vi "Write mode ref.vi"(8 "error in (no error)":errorcluster caption="에러 입력(에러 없음)", 10 "mode ref":refnum<vi>, 11 "Haptic IC 입력":refnum<class "Haptic IC.lvclass">) -> (0 "error out":errorcluster caption="에러 출력", 3 "Haptic IC 출력":refnum<class "Haptic IC.lvclass">)   [LabVIEW 2020, in "Haptic IC.lvclass"]
uses:
  Haptic IC.lvclass
  Haptic IC.lvclass/Haptic IC.ctl
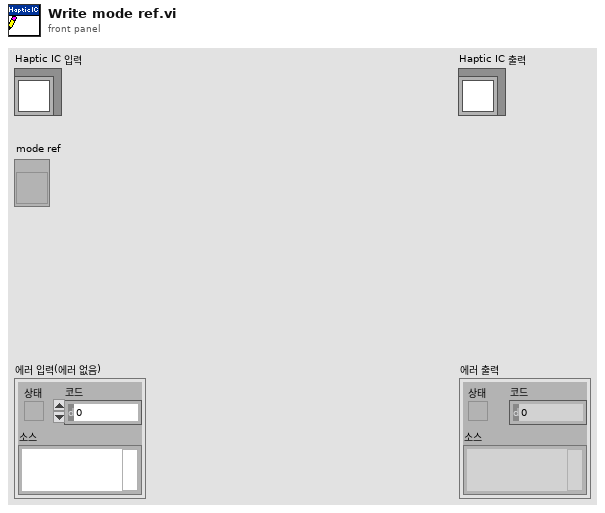
[diagram p1: front panel]
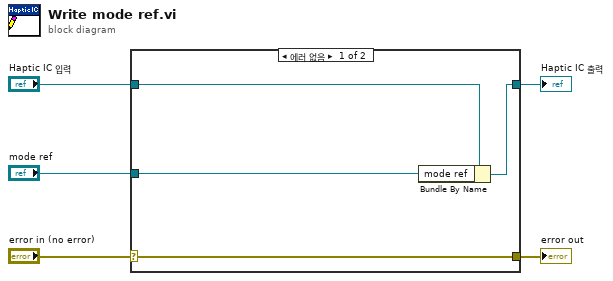
[diagram p0: block diagram]
diagram:
  n1 = case shown="에러 없음" "error in (no error)" {
    selector: "error in (no error)" -> [w9 w10]
    tunnel: [w9 w10] -> w4
    tunnel: [w7 w11] -> w2
    tunnel: "Haptic IC 입력" -> [w8 w11]
    tunnel: "mode ref" -> [w6 _]
    frame No Error {
      n2 = Bundle By Name(cluster=w8, "mode ref"=w6) -> (w7:refnum<class "Haptic IC.lvclass">)
    }
    frame Error {
    }
  }
  "error out" <- w4
  "Haptic IC 출력" <- w2
